vi "MQTT_Q_Disconnect.vi"(8 "error in (no error)":errorcluster, 11 "MQTT_Q In":refnum<class "MQTT_Q.lvclass">) -> (0 "error out":errorcluster)   [LabVIEW 2015, in "MQTT_Q.lvclass"]
uses:
  MQTT_Q.lvclass
  MQTT_Q_PVT_MessageType.ctl
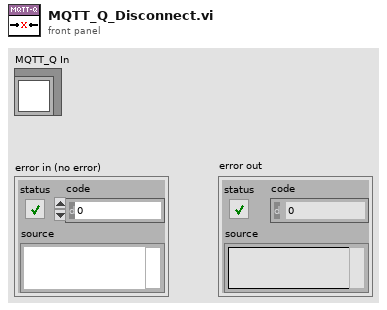
[diagram p1: front panel]
types:
  T1 = typedef "MQTT_Q.lvclass/MQTT_Q_PVT_MessageType.ctl" = enum32{"Reserved", "CONNECT", "CONNACK", "PUBLISH", "PUBACK", "PUBREC", "PUBREL", "PUBCOMP", "SUBSCRIBE", "SUBACK", "UNSUBSCRIBE", "UNSUBACK", "PINGREQ", "PINGRESP", "DISCONNECT", "Reserved2"}
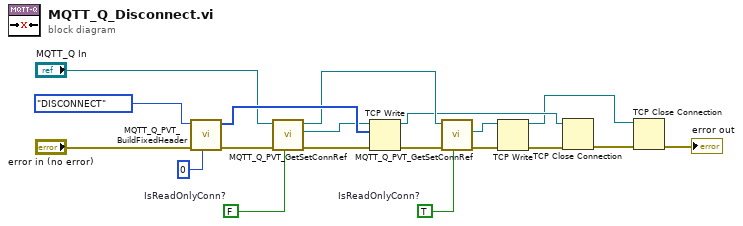
[diagram p0: block diagram]
diagram:
  w1 = FALSE  # IsReadOnlyConn?
  w2 = TRUE  # IsReadOnlyConn?
  n1 = call "MQTT_Q_PVT_BuildFixedHeader.vi"("Remaining Length"=u32 0, "error in (no error)"="error in (no error)", "MessageType"=MQTT_Q_PVT_MessageType."DISCONNECT") -> ("error out"=w13:errorcluster, "Fixed Header"=w16:u8[])  [unwired: 7 in]
  n2 = call "MQTT_Q_PVT_GetSetConnRef.vi"("IsReadOnlyConn?"=w1, "error in (no error)"=w13, "MQTT_Q in"="MQTT_Q In") -> ("error out"=w12:errorcluster, "connection ID Out"=w11:refnum<k5>, "MQTT_Q out"=w9:refnum<class "MQTT_Q.lvclass">)  [unwired: 6 in]
  n3 = TCP Write(connection ID=w11, data in=w16, error in (no error)=w12) -> (connection ID out=w4:refnum<k5>, error out=w10:errorcluster)  [unwired: 1 in, 1 out]
  n4 = call "MQTT_Q_PVT_GetSetConnRef.vi"("IsReadOnlyConn?"=w2, "error in (no error)"=w10, "MQTT_Q in"=w9) -> ("error out"=w8:errorcluster, "connection ID Out"=w7:refnum<k5>)  [unwired: 6 in, 1 out]
  n5 = TCP Write(connection ID=w7, error in (no error)=w8) -> (connection ID out=w3:refnum<k5>, error out=w6:errorcluster)  [unwired: 2 in, 1 out]
  n6 = TCP Close Connection(connection ID=w4, error in (no error)=w6) -> (error out=w5:errorcluster)  [unwired: 1 in, 1 out]
  n7 = TCP Close Connection(connection ID=w3, error in (no error)=w5) -> (error out=→"error out":errorcluster)  [unwired: 1 in, 1 out]
